vi "Set Control Value.vi"(8 "error in (no error)":errorcluster, 10 "Value":variant, 11 "Ctl Refnum":refnum<vi>) -> (0 "error out":errorcluster, 3 "Ctl Refnum out":refnum<vi>)   [LabVIEW 2017, in "UI Common.lvlib"]
uses:
  UI Common.lvlib
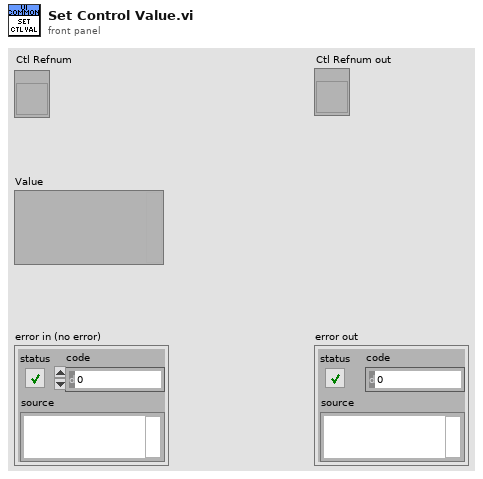
[diagram p1: front panel]
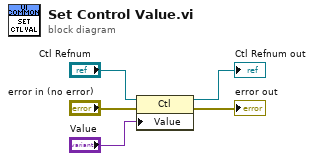
[diagram p0: block diagram]
diagram:
  n1 = property class="Ctl"(reference="Ctl Refnum", error in="error in (no error)", "Value"="Value") -> (reference out=→"Ctl Refnum out":refnum<vi>, error out=→"error out":errorcluster)
